vi "Lab3_FSK2.vi"() -> ()   [LabVIEW 2019]
uses:
  <vilib>/addons/Modulation/Digital/General/MT Generate Bits (Galois, PN Order).vi
  <vilib>/addons/Modulation/Analog/support/mod_Set Error Source.vi
  <vilib>/addons/Modulation/Digital/Support/Common/Validators/mod_Generate Bits Validate.vi
  <vilib>/addons/Modulation/Digital/Support/Common/Validators/mod_AWGN Validate.vi
  <vilib>/addons/Modulation/Digital/Impairments/subVIs/mod_createSeeds.vi
  <vilib>/addons/Modulation/Digital/Support/Common/Validators/mod_Validate Samples Per Symbol.vi
  <vilib>/addons/Modulation/Analog/support/Validators/mod_Validate Complex Waveform.vi
  <vilib>/addons/Modulation/Analog/support/Validators/mod_WFErrorHandler.vi
  <vilib>/addons/Modulation/Digital/General/MT Generate FSK System Parameters(M).vi
  <vilib>/addons/Modulation/Digital/General/subVIs/mod_Generate Bits PN Sequence.vi
  <vilib>/Analysis/1siggen.llb/Gaussian White Noise (obs 90).vi
  <vilib>/addons/Modulation/Analog/MT Upconvert Baseband (Real).vi
  <vilib>/express/express analysis/Spectral/Block/exnSpectralBlock spectral measurements RMS poly.vi
  <vilib>/express/express analysis/Spectral/Block/exnSpectralBlock spectral measurements RMS DDT.vi
  <vilib>/addons/Modulation/Digital/Support/Common/Validators/mod_Generate Filter Coefficients Validate.vi
  <vilib>/addons/Modulation/Digital/General/subVIs/mod_Generate Filter Coefficients.vi
  <vilib>/express/express analysis/Spectral/XNode/ExpressSpectralMeasurementsBlockNode.xnode
  <vilib>/addons/Modulation/niDMT.lvlib
  <vilib>/addons/Modulation/niAMT.lvlib
panel:
  in  "Eb/No(dB)":dbl
  in  "FSK Derivation(Hz)":dbl format="%#_2p"
  in  "Symbol(Hz) Rate(HZ)":dbl format="%#_2p"
  in  "pulse shaping filter (none)":T1(ring)
  in  "Carrier Freq(HZ)":dbl format="%#_2p"
  in  "M-FSK":u16(ring) items=["2"=2, "4"=4, "8"=8, "16"=16]
  in  "stop":bool
  in  "Tab Control":T2(tab)
  out "FFT-RMS":dynamicdata(graph)
  out "Modulated Signal(Passband)":waveform(dbl)(graph)
  out "ch_in":cluster{"t0":dbl, "dt":dbl, "Y":dbl[]}(graph)
  out "ch_out":cluster{"t0":dbl, "dt":dbl, "Y":dbl[]}(graph)
  # "M-FSK"
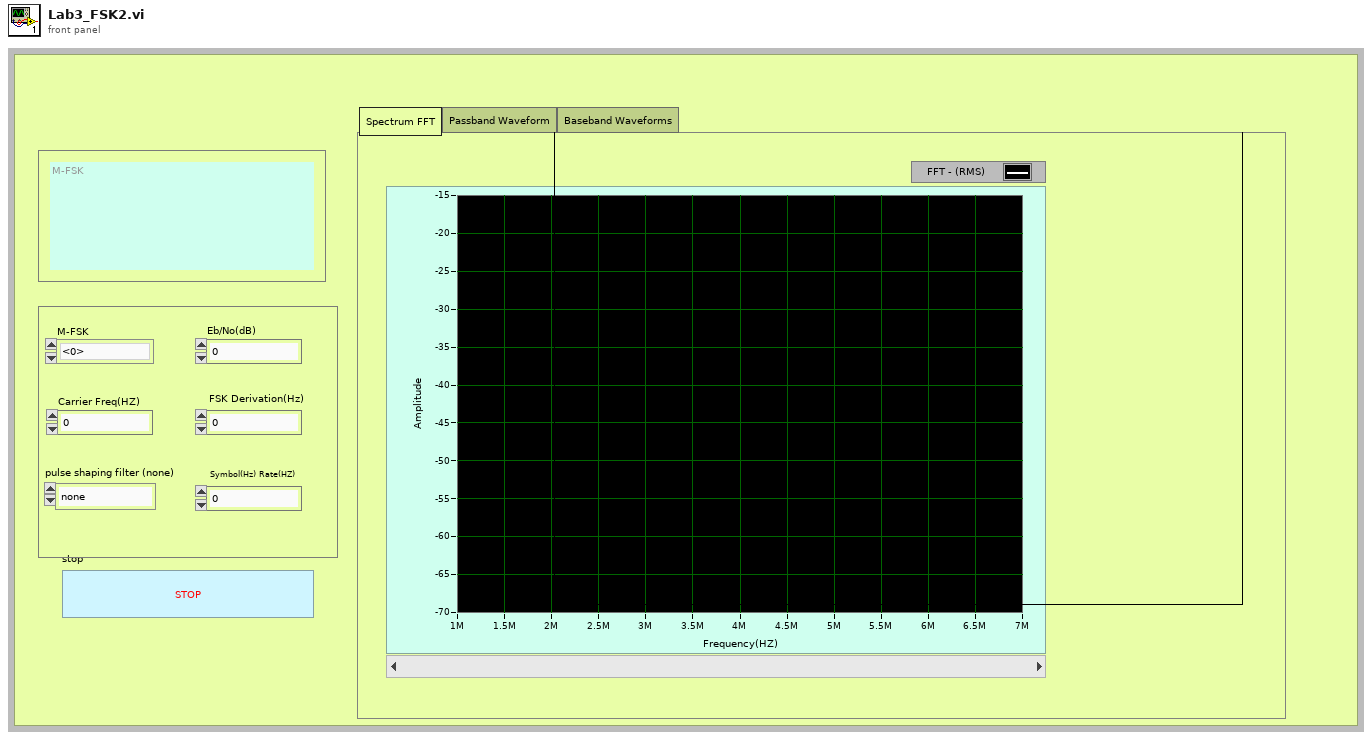
[diagram p1: front panel]
types:
  T1 = enum16{"none", "Raised Cosine", "Root Raised Cos", "Gaussian"}
  T2 = enum32{"Spectrum FFT", "Passband Waveform", "Baseband Waveforms"}
  T3 = enum16{"FSK", "PSK", "QAM", "MSK", "PAM", "ASK", "CPM"}
  T4 = cluster{"averaging mode":u16, "weighting mode":u16, "number of averages":u32}
  T5 = cluster{"dB On (F)":bool, "unwrap phase (F)":bool, "convert to degree (F)":bool}
  T6 = cluster{"samples per symbol (16)":i32, "symbol map":dbl[], "symbol phase continuity":enum16{"continuous", "discontinuous"}}
  T7 = typedef "niAMT.lvlib/Complex Data Waveform.ctl" = cluster{"t0":dbl, "dt":dbl, "Y":cdb[]}
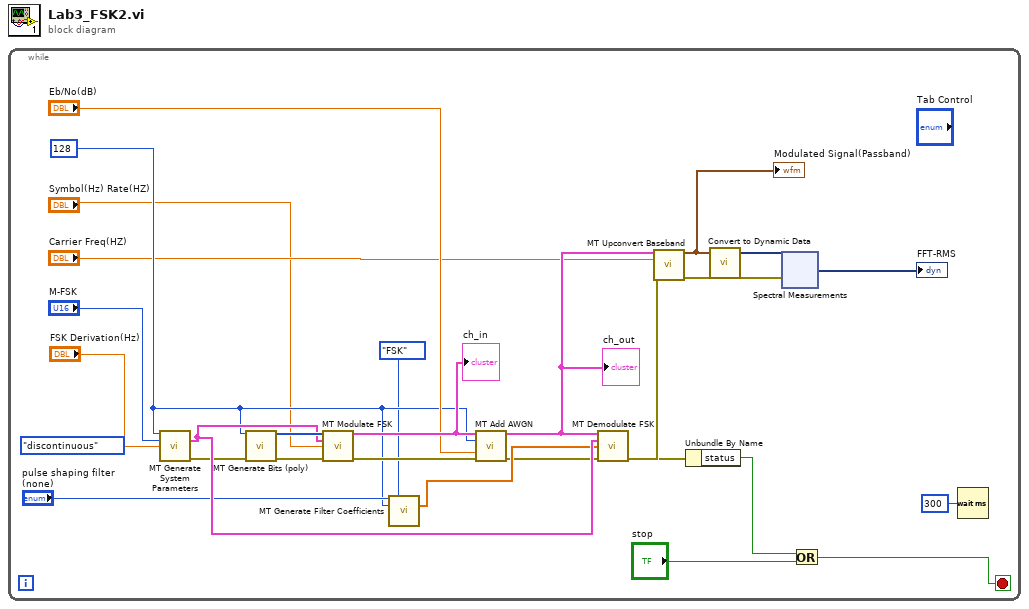
[diagram p0: block diagram]
diagram:
  n1 = while {
    stop <- w1 stop-if-true
    w15 = 128
    n2 = call-poly <vilib>:"MT Generate System Parameters.vi"("samples per symbol (16)"=w15, "M-FSK (2)"="M-FSK", "FSK deviation (Hz)"="FSK Derivation(Hz)", "symbol phase continuity"=enum16{"continuous", "discontinuous"}."discontinuous") -> ("FSK system parameters"=w25:T6, "error out"=w19:errorcluster)  [unwired: 9 in, 1 out]
    n3 = call-poly <vilib>:"MT Generate Bits (poly).vi"("total bits (128)"=w15, "error in (no error)"=w19) -> ("output bit stream"=w26:i8[], "error out"=w18:errorcluster)  [unwired: 11 in, 1 out]
    n4 = call <vilib>:"MT Modulate FSK.vi"("input bit stream"=w26, "FSK system parameters"=w25, "symbol rate (Hz)"="Symbol(Hz) Rate(HZ)", "error in (no error)"=w18) -> ("output complex waveform"=w20:T7, "error out"=w17:errorcluster)  [unwired: 9 in, 1 out]
    "ch_in" <- w20
    n5 = call <vilib>:"MT Generate Filter Coefficients.vi"("pulse shaping filter (none)"="pulse shaping filter (none)", "modulation type"=T3."FSK", "pulse shaping samples per symbol (16)"=w15) -> ("matched filter coefficients"=w24:dbl[])  [unwired: 10 in, 2 out]
    n6 = call <vilib>:"MT Add AWGN.vi"("input complex waveform"=w20, "samples per symbol (16)"=w15, "Eb/N0 (10 dB)"="Eb/No(dB)", "error in (no error)"=w17) -> ("output complex waveform"=w23:T7, "error out"=w21:errorcluster)  [unwired: 9 in, 1 out]
    "ch_out" <- w23
    n7 = call <vilib>:"MT Demodulate FSK.vi"("input complex waveform"=w23, "FSK system parameters"=w25, "matched filter coefficients"=w24, "error in (no error)"=w21) -> ("error out"=w14:errorcluster)  [unwired: 7 in, 4 out]
    n8 = call-poly <vilib>:"MT Upconvert Baseband.vi"("baseband waveform (complex)"=w23, "carrier frequency (Hz)"="Carrier Freq(HZ)", "error in (no error)"=w21) -> ("passband waveform"=w13:waveform(dbl), "error out"=w5:errorcluster)  [unwired: 11 in]
    "Modulated Signal(Passband)" <- w13
    n9 = Unbundle By Name(w14) -> ("status"=w11:bool)
    n10 = call "Convert to Dynamic Data"("Waveform"=w13) -> ("Dynamic Data Type"=w4:dynamicdata)  [unwired: 3 in]
    n11 = xnode "Spectral Measurements"("Signals"=w4, "error in (no error)"=w5) -> ("FFT - (RMS)"=→"FFT-RMS":dynamicdata)  [unwired: 2 out]
    n12 = Or(x=w11, y="stop") -> (x .or. y?=w1:bool)
    n13 = Wait (ms)(milliseconds to wait=u32 300) -> ()  [unwired: 1 out]
  }
